vi "flatten (i16 2d).vi"(3 "array":i16[][](array[numeric])) -> (1 "flattened":i16[](array[numeric]))   [LabVIEW 2012, in "common.lvlib"]
uses:
  common.lvlib
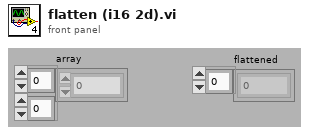
[diagram p1: front panel]
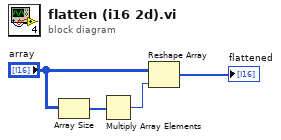
[diagram p0: block diagram]
diagram:
  n1 = Array Size(array="array") -> (size(s)=w4:i32[])
  n2 = Multiply Array Elements(1:w4) -> (0:w2:i32)
  n3 = Reshape Array("array", w2) -> (→"flattened":i16[])
